vi "soulpaser.vi"(11 "rionav?":bool) -> ()   [LabVIEW 2015]
uses:
  G_NAV.vi
  G_VEH.vi
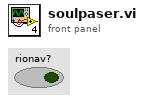
[diagram p1: front panel]
types:
  T1 = enum16{"big-endian, network order", "native, host order", "little-endian"}
  T2 = cluster{"GPSTime":dbl, "accel[0]":sgl, "accel[1]":sgl, "accel[2]":sgl, "pqr[0]":sgl, "pqr[1]":sgl, "pqr[2]":sgl, "llh[0]":dbl, "llh[1]":dbl, "llh[2]":dbl, "vel_ned[0]":sgl, "vel_ned[1]":sgl, "vel_ned[2]":sgl, "attitude[0]":sgl, "attitude[1]":sgl, "attitude[2]":sgl, "vel_bxyz[0]":sgl, "vel_bxyz[1]":sgl, "vel_bxyz[2]":sgl, "lcc[0]":sgl, "lcc[1]":sgl, "lcc[2]":sgl, "CovKalman[0]":sgl, "CovKalman[1]":sgl, "CovKalman[2]":sgl, "CovKalman[3]":sgl, "CovKalman[4]":sgl, "CovKalman[5]":sgl, "llh_GPS[0]":sgl, "llh_GPS[1]":sgl, "llh_GPS[2]":sgl, "vel_GPS[0]":sgl, "vel_GPS[1]":sgl, "vel_GPS[2]":sgl, "heading_Magnetic":sgl, "heading_GPS":sgl, "GPSStatus":u16, "FailureCode":u16, "DataChecksum":u16}
  T3 = cluster{"sop1":u8, "sop2":u8, "sop3":u8, "header_length":u8, "number":u16, "type":u8, "port_address":u8, "length":u16, "sequence":u16, "idle":u8, "gps_stat":u8, "gps_week":u16, "millisecs":u32, "status":u32, "crc":u16, "version":u16}
  T4 = cluster{"sol_stat":u32, "pos_type":u32, "lat":dbl, "lon":dbl, "hgt":dbl, "und":sgl, "datum_id":i32, "latdev":sgl, "londev":sgl, "hgtdev":sgl, "ref_station_id 0":i8, "ref_station_id 1":i8, "ref_station_id 2":i8, "ref_station_id 3":i8, "lag":sgl, "age":sgl, "sats":u8, "gps_l1_ranges":u8, "gps_l1_mask_ranges":u8, "gps_l2_mask_ranges":u8, "reserved":i8, "ext_sol_stat":u8, "reserved2":u8, "sig_mask":u8}
  T5 = cluster{"Steer_input":dbl, "Steer_output":dbl, "VS_des":dbl, "VS_can":dbl, "heading":dbl, "auto":bool, "run":bool, "x":dbl, "y":dbl}
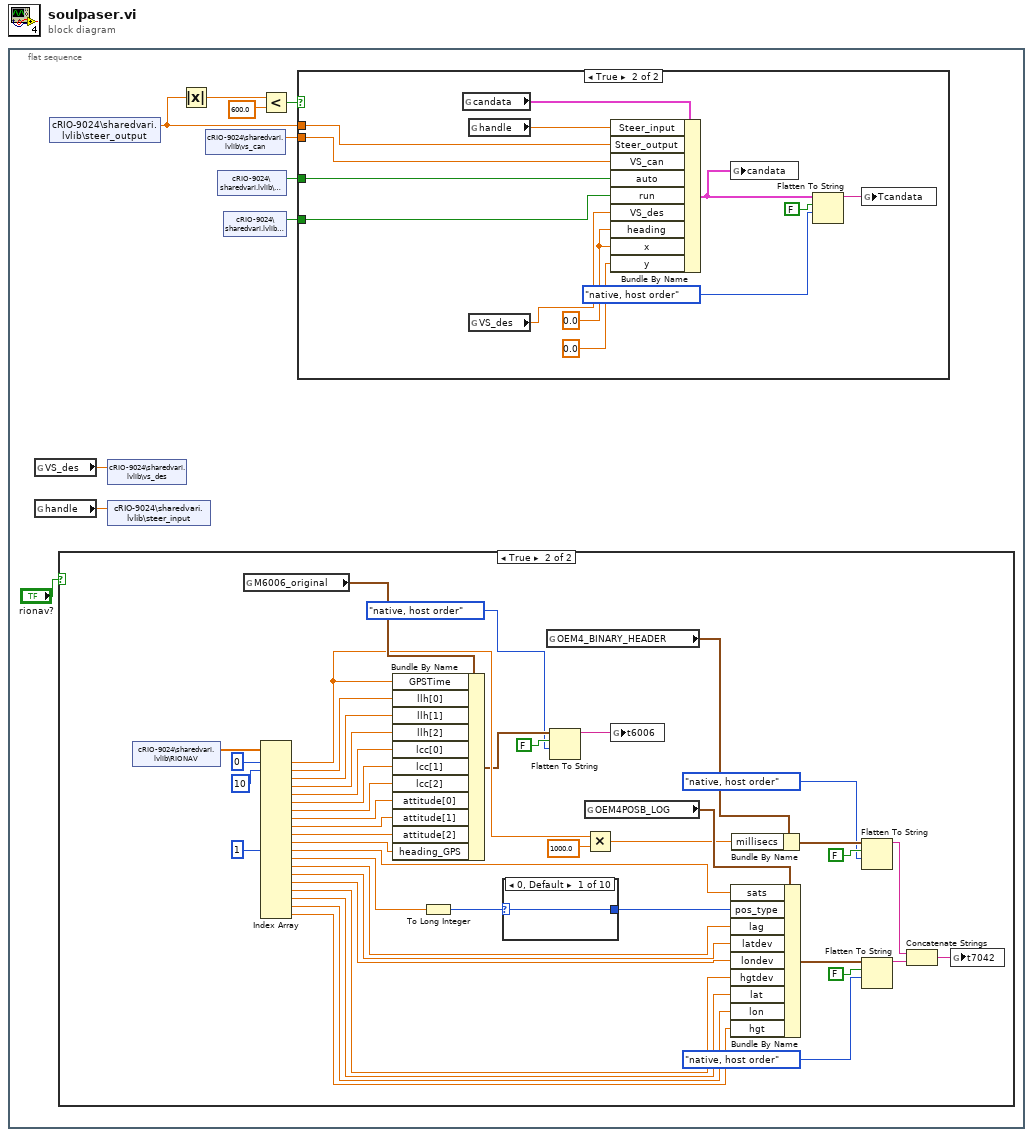
[diagram p0: block diagram]
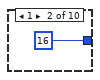
[diagram p3: hidden frame]
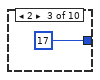
[diagram p4: hidden frame]
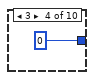
[diagram p5: hidden frame]
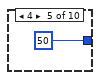
[diagram p6: hidden frame]
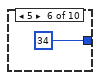
[diagram p7: hidden frame]
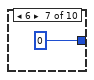
[diagram p8: hidden frame]
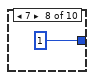
[diagram p9: hidden frame]
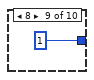
[diagram p10: hidden frame]
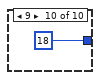
[diagram p11: hidden frame]
diagram:
  n1 = flat-sequence {
    frame #0 {
      n2 = global read "G_VEH.vi" "VS_des"() -> (w6:dbl)
      n3 = global read "G_VEH.vi" "handle"() -> (w3:dbl)
      n4 = shared-variable "cRIO-9024\\sharedvari.lvlib\\steer_output"() -> (w7:dbl)  [unwired: 1 in, 1 out]
      n5 = case shown="True" "rionav?" {
        frame False {
        }
        frame True {
          n6 = shared-variable "cRIO-9024\\sharedvari.lvlib\\RIONAV"() -> (w54:dbl[])  [unwired: 1 in, 1 out]
          n7 = global read "G_NAV.vi" "M6006_original"() -> (w52:T2)
          n8 = Index Array(array=w54, index #1=0 ("index"), index #2=10 ("index"), index #12=1 ("index")) -> (element #1=w40:dbl, element #2=w50:dbl, element #3=w49:dbl, element #4=w48:dbl, element #5=w13:dbl, element #6=w12:dbl, element #7=w47:dbl, element #8=w46:dbl, element #9=w45:dbl, element #10=w11:dbl, element #11=w16:dbl, element #12=w18:dbl, element #13=w19:dbl, element #14=w20:dbl, element #15=w21:dbl, element #16=w22:dbl, element #17=w23:dbl, element #18=w15:dbl, element #19=w14:dbl, element #20=w24:dbl)  [unwired: 17 in]
          n9 = Bundle By Name(cluster=w52, "GPSTime"=w40, "llh[0]"=w50, "llh[1]"=w49, "llh[2]"=w48, "lcc[0]"=w13, "lcc[1]"=w12, "lcc[2]"=w47, "attitude[0]"=w46, "attitude[1]"=w45, "attitude[2]"=w11, "heading_GPS"=w16) -> (w37:T2)
          n10 = To Long Integer(number=w19) -> (32bit integer=w43:i32)
          n11 = case shown="0, Default" w43 {
            selector: w43 -> [w55 _ _ _ _ _ _ _ _ _]
            tunnel: [w55 16 17 0 50 34 0 1 1 18] -> w42
            frame 0, Default {
            }
            frame 1 {
            }
            frame 2 {
            }
            frame 3 {
            }
            frame 4 {
            }
            frame 5 {
            }
            frame 6 {
            }
            frame 7 {
            }
            frame 8 {
            }
            frame 9 {
            }
          }
          n12 = global read "G_NAV.vi" "OEM4_BINARY_HEADER"() -> (w41:T3)
          n13 = Flatten To String(anything=w37, prepend array or string size? (T)=FALSE, byte order (0:big-endian, network order)=T1."native, host order") -> (data string=w34:string)  [unwired: 1 in, 2 out]
          n14 = global read "G_NAV.vi" "OEM4POSB_LOG"() -> (w44:T4)
          n15 = Multiply(x=w40, y=1000.0) -> (x*y=w38:dbl)
          n16 = global write "G_NAV.vi" "t6006"(w34) -> ()
          n17 = Bundle By Name(cluster=w44, "sats"=w18, "pos_type"=w42, "lag"=w20, "latdev"=w21, "londev"=w22, "hgtdev"=w23, "lat"=w15, "lon"=w14, "hgt"=w24) -> (w28:T4)
          n18 = Bundle By Name(cluster=w41, "millisecs"=w38) -> (w32:T3)
          n19 = Flatten To String(anything=w32, prepend array or string size? (T)=FALSE, byte order (0:big-endian, network order)=T1."native, host order") -> (data string=w27:string)  [unwired: 1 in, 2 out]
          n20 = Flatten To String(anything=w28, prepend array or string size? (T)=FALSE, byte order (0:big-endian, network order)=T1."native, host order") -> (data string=w26:string)  [unwired: 1 in, 2 out]
          n21 = Concatenate Strings(w27, w26) -> (w25:string)
          n22 = global write "G_NAV.vi" "t7042"(w25) -> ()
        }
      }
      n23 = shared-variable "cRIO-9024\\sharedvari.lvlib\\vs_des"(w6) -> ()  [unwired: 1 in, 1 out]
      n24 = shared-variable "cRIO-9024\\sharedvari.lvlib\\steer_input"(w3) -> ()  [unwired: 1 in, 1 out]
      n25 = Absolute Value(x=w7) -> (abs(x)=w10:dbl)
      n26 = shared-variable "cRIO-9024\\sharedvari.lvlib\\vs_can"() -> (w2:dbl)  [unwired: 1 in, 1 out]
      n27 = shared-variable "cRIO-9024\\sharedvari.lvlib\\auto"() -> (w5:bool)  [unwired: 1 in, 1 out]
      n28 = shared-variable "cRIO-9024\\sharedvari.lvlib\\run"() -> (w4:bool)  [unwired: 1 in, 1 out]
      n29 = Less?(x=w10, y=600.0) -> (x < y?=w8:bool)
      n30 = case shown="True" w8 {
        tunnel: w7 -> [_ w77]
        tunnel: w5 -> [_ w70]
        tunnel: w4 -> [_ w69]
        tunnel: w2 -> [_ w71]
        frame False {
        }
        frame True {
          w66 = 0.0 ("x")
          n31 = global read "G_VEH.vi" "candata"() -> (w72:T5)
          n32 = global read "G_VEH.vi" "handle"() -> (w65:dbl)
          n33 = global read "G_VEH.vi" "VS_des"() -> (w68:dbl)
          n34 = Bundle By Name(cluster=w72, "Steer_input"=w65, "Steer_output"=w77, "VS_can"=w71, "auto"=w70, "run"=w69, "VS_des"=w68, "heading"=w66, "x"=w66, "y"=0.0) -> (w76:T5)
          n35 = global write "G_VEH.vi" "candata"(w76) -> ()
          n36 = Flatten To String(anything=w76, prepend array or string size? (T)=FALSE, byte order (0:big-endian, network order)=T1."native, host order") -> (data string=w73:string)  [unwired: 1 in, 2 out]
          n37 = global write "G_VEH.vi" "Tcandata"(w73) -> ()
        }
      }
    }
  }
